vi "Get Color Example.vi"() -> ()   [LabVIEW 2018, in "ColorSensor.lvlib"]
uses:
  ColorSensor.lvlib
  TypeDef/Color.ctl
panel:
  out "Detected Color":T1
  out "Confidence":dbl
  in  "Confidence Threshold":dbl=0.95
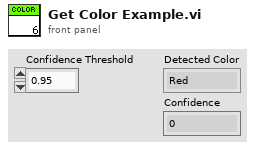
[diagram p1: front panel]
types:
  T1 = typedef "ColorSensor.lvlib/Color.ctl" = enum16{"Red", "Green", "Blue", "Yellow", "Unknown"}
  T2 = typedef "ColorSensor.lvlib/ColorSensorDevRef.ctl" = cluster{"I2CDevRef":T3, "Confidence Threshold":dbl}
  T3 = typedef "WPI_I2CDevRef.ctl" = cluster{"DevStatus":errorcluster, "Device Address":u8, "Handle":i32, "I2C Bus":T4}
  T4 = typedef "i2c_bus.ctl" = enum16{"I2C On-Board", "I2C MXP", "Invalid"}
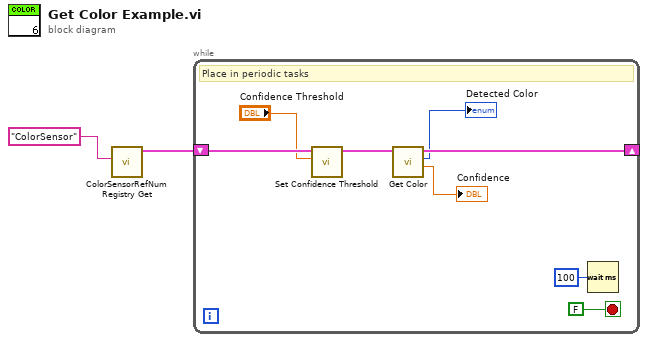
[diagram p0: block diagram]
diagram:
  n1 = call "ColorSensorRefNum Registry Get.vi"("refnum name"="ColorSensor") -> ("ColorSensorDevRef"=w1:T2)  [unwired: 9 in, 1 out]
  n2 = while {
    shift-right: [w8] -> _
    shift-left: w1 -> [w5]
    stop <- FALSE stop-if-true
    # "Place in periodic tasks"
    n3 = call "Set Confidence Threshold.vi"("Confidence Threshold"="Confidence Threshold", "ColorSensorDevRef"=w5) -> ("ColorSensorDevRef out"=w4:T2)  [unwired: 8 in, 1 out]
    n4 = call "Get Color.vi"("ColorSensorDevRef"=w4) -> ("Confidence"=→"Confidence":dbl, "Color"=→"Detected Color":T1, "ColorSensorDevRef out"=w8:T2)  [unwired: 7 in, 1 out]
    n5 = Wait (ms)(milliseconds to wait=u32 100) -> ()  [unwired: 1 out]
  }
